vi "MGI Test Cluster Index.vi"() -> ()   [LabVIEW 2016]
panel:
  in  "Inputs":string[](array[string])=["I32", "DBL", "String", "Cluster", "SGL", "Sub-str", "Bool", "Enum"]
  out "Results":i32[](array[numeric])
  in  "Mode":T1(ring)
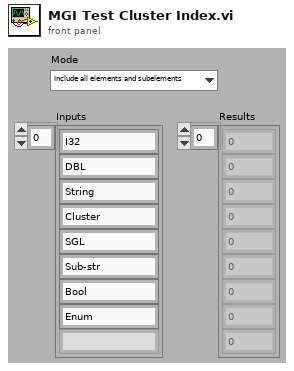
[diagram p1: front panel]
types:
  T1 = enum16{"Include all elements and subelements", "First level only", "Index in lowest level"}
  T2 = cluster{"I32":i32, "DBL":dbl, "String":string, "Cluster":cluster{"SGL":sgl, "Sub-str":string, "blah 0":i32, "blah 1":i32, "blah 2":i32, "blah 3":i32}, "Bool":bool, "Enum":enum16{"A", "B", "C"}}
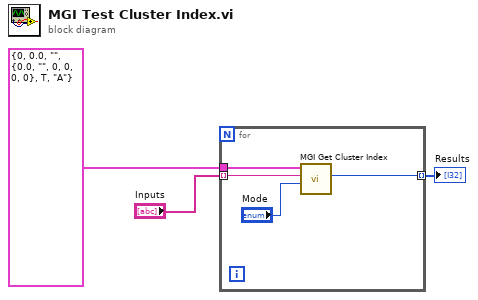
[diagram p0: block diagram]
diagram:
  n1 = for {
    tunnel: T2 {"I32"=0, "DBL"=0.0, "String"="", "Cluster"={"SGL"=0.0, "Sub-str"="", "blah 0"=0, "blah 1"=0, "blah 2"=0, "blah 3"=0}, "Bool"=TRUE, "Enum"=enum."A"} -> [w7]
    tunnel: "Inputs" -> [w6] mode=indexing
    tunnel: [w4] -> w1 mode=indexing
    n2 = call <userlib>:"MGI Get Cluster Index.vi"("Mode"="Mode", "Name"=w6, "Cluster In"=w7) -> ("Index"=w4:i32)  [unwired: 7 in, 1 out]
  }
  "Results" <- w1
